vi "Taiko_ErrorDlg.vi"(8 "Error in":errorcluster) -> (0 "Error":errorcluster, 3 "Exit":bool)   [LabVIEW 2010]
panel:
  in  "Exit":bool
  in  "Ignore":bool
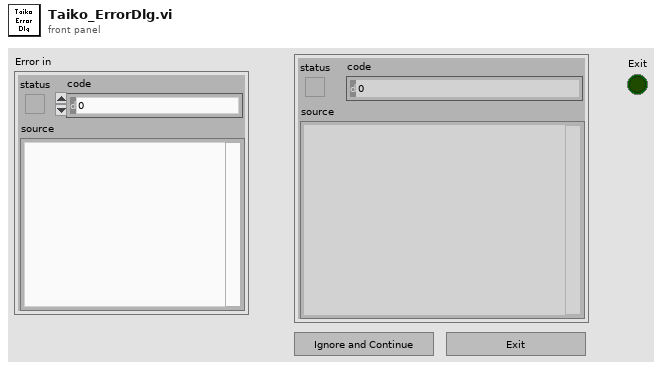
[diagram p1: front panel]
types:
  T1 = enum32{"Invalid", "Standard", "Closed", "Hidden", "Minimized", "Maximized"}
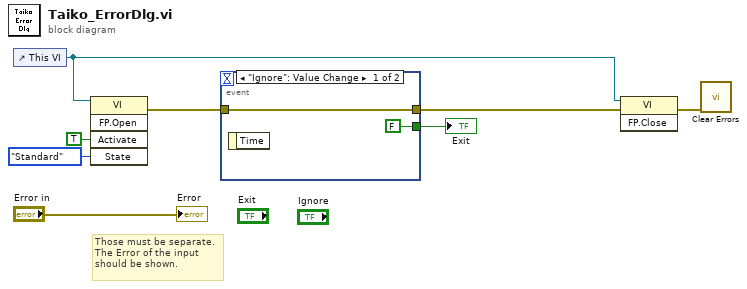
[diagram p0: block diagram]
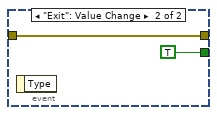
[diagram p2: hidden frame]
diagram:
  # "Those must be separate.\nThe Error of the input\nshould be shown."
  n1 = control-ref of="This VI"() -> (w4:refnum<vi>)
  n2 = invoke class="VI" method="FP.Open"(reference=w4, "Activate"=TRUE ("Activate?"), "State"=T1."Standard") -> (error out=w3:errorcluster)  [unwired: 2 in, 4 out]
  n3 = event shown="[0] \"Ignore\": Value Change" {
    selector: _ -> [_ _]
    dyn-events: _ -> [_ _]
    timeout: _ -> [_ _]
    tunnel: w3 -> [w9 w11]
    tunnel: [FALSE TRUE] -> w6
    tunnel: [w9 w11] -> w5
    event "Ignore": Value Change {
      n4 = event-data() -> ()  [unwired: 1 in, 1 out]
    }
    event "Exit": Value Change {
      n5 = event-data() -> ()  [unwired: 1 in, 1 out]
    }
  }
  "Exit" <- w6
  n6 = invoke class="VI" method="FP.Close"(reference=w4, error in=w5) -> (error out=w1:errorcluster)  [unwired: 1 in, 2 out]
  n7 = call <vilib>:"Clear Errors.vi"("error in (no error)"=w1) -> ()  [unwired: 5 in, 2 out]
  "Error" <- "Error in"
